vi "open Subscriber connection.vi"(4 "error in (no error)":errorcluster, 5 "Machine":string="192.168.10.182", 6 "Port":u16=64535, 7 "Subscriber list":string="opticalspectrum") -> (0 "error out":errorcluster, 3 "connection ID":refnum<k5>)   [LabVIEW 2013]
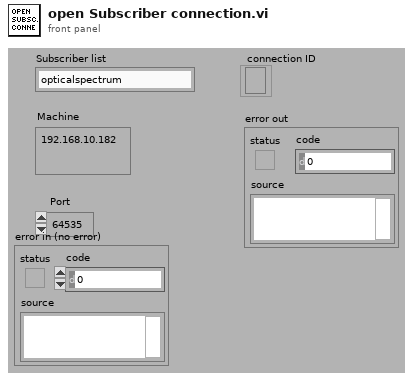
[diagram p1: front panel]
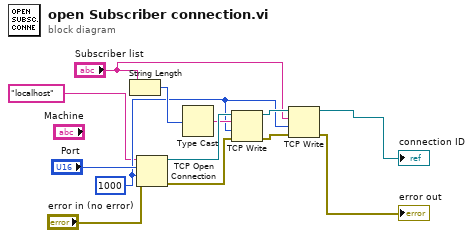
[diagram p0: block diagram]
diagram:
  w2 = 1000 ("timeout ms (60000)")
  n1 = String Length(string="Subscriber list") -> (length=w5:i32)
  n2 = TCP Open Connection(address="localhost" ("Machine"), remote port or service name="Port", timeout ms (60000)=w2, error in (no error)="error in (no error)") -> (connection ID=w8:refnum<k5>, error out=w11:errorcluster)  [unwired: 1 out]
  n3 = Type Cast(x=w5) -> (*(type *) &x=w6:string)  [unwired: 1 in]
  n4 = TCP Write(connection ID=w8, data in=w6, error in (no error)=w11, 9:w2) -> (connection ID out=w9:refnum<k5>, error out=w10:errorcluster)  [unwired: 1 out]
  n5 = TCP Write(connection ID=w9, data in="Subscriber list", error in (no error)=w10, 9:w2) -> (connection ID out=→"connection ID":refnum<k5>, error out=→"error out":errorcluster)  [unwired: 1 out]
